vi "create digital output command.vi"(9 "new output":bool, 10 "module":enum16{"7", "8"}(ring), 11 "Index":i32) -> (3 "command message":variant)   [LabVIEW 2018]
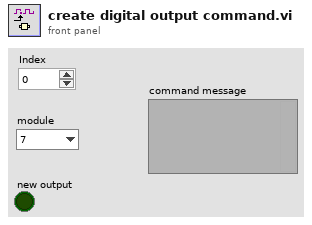
[diagram p1: front panel]
types:
  T1 = cluster{"new output":bool, "module":enum16{"7", "8"}, "Index":i32}
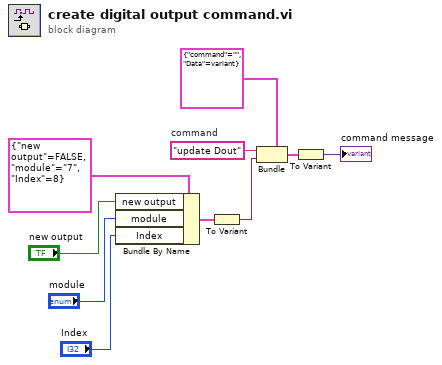
[diagram p0: block diagram]
diagram:
  w7 = "update Dout"  # command
  n1 = Bundle By Name(cluster=T1 {"new output"=FALSE, "module"=enum."7", "Index"=8}, "new output"="new output", "module"="module", "Index"="Index") -> (w9:T1)
  n2 = To Variant(anything=w9) -> (Variant=w6:variant)
  n3 = Bundle(cluster=cluster{"command":string, "Data":variant} {"command"="", "Data"=variant}, "command"=w7, "Data"=w6) -> (w5:cluster{"command":string, "Data":variant})
  n4 = To Variant(anything=w5) -> (Variant=→"command message":variant)
